vi "build ID byte.vi"(8 "Output?":bool, 9 "Input?":bool, 10 "Node ID":dbl, 11 "Type":u16(ring) items=["Central node", "Portable control", "Boolean sensor", "Boolean output", "8-bit sensor", "8-bit output"]) -> (2 "ID byte":string, 3 "Boolean array":bool[](array[boolean]))   [LabVIEW 2011]
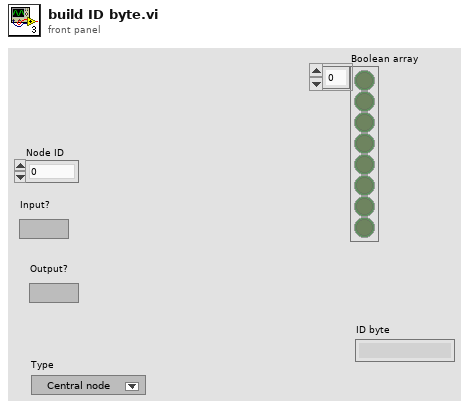
[diagram p1: front panel]
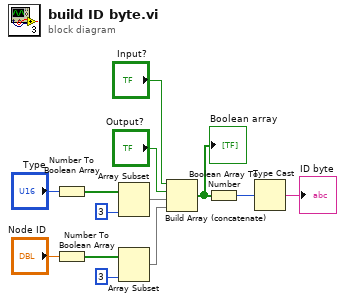
[diagram p0: block diagram]
diagram:
  n1 = Number To Boolean Array(number="Type") -> (Boolean array=w9:bool[])
  n2 = Number To Boolean Array(number="Node ID") -> (Boolean array=w5:bool[])
  n3 = Array Subset(array=w9, length=3) -> (w7:bool[])  [unwired: 1 in]
  n4 = Array Subset(array=w5, length=3) -> (w4:bool[])  [unwired: 1 in]
  n5 = Build Array (concatenate)("Input?", "Output?", w7, w4) -> (w3:bool[])
  "Boolean array" <- w3
  n6 = Boolean Array To Number(Boolean array=w3) -> (number=w2:u32)
  n7 = Type Cast(x=w2) -> (*(type *) &x=→"ID byte":string)  [unwired: 1 in]
